vi "Read_Write_Plot_Setup.vi"(6 "jobDirectory":path, 7 "Mode":enum16{"Load", "Save"}(ring), 9 "Setup filename":string, 11 "Cluster":T1={"Result files to read"=[], "Template"=path "", "Transpose"=FALSE, "Additional X Values"=[], "Additional Y Values"=[], "Output Filename"=path "", "Create Picture Vi Name"="Intensity plot jpg.vi", "Intensity Plot?"=FALSE, "Multi Ordinate"=[], "Abscissa String"="", "Filter Array"=["", "", "", "", "", ""], "Filter Bins 1 Strings"=[""], "Filter Bins 2 Strings"=[""], "Filters 3 onwards"=[], "nRows"=0} {"Additional Y Values" format="%.2f"; "Additional X Values" format="%.2f"}) -> (0 "OK?":bool, 1 "setupLoaded":path, 3 "Cluster 2":T1={"Result files to read"=[], "Template"=path "", "Transpose"=FALSE, "Additional X Values"=[], "Additional Y Values"=[], "Output Filename"=path "", "Create Picture Vi Name"="Intensity plot jpg.vi", "Intensity Plot?"=FALSE, "Multi Ordinate"=[], "Abscissa String"="", "Filter Array"=["", "", "", "", "", ""], "Filter Bins 1 Strings"=[""], "Filter Bins 2 Strings"=[""], "Filters 3 onwards"=[], "nRows"=0} {"Additional Y Values" format="%.2f"; "Additional X Values" format="%.2f"})   [LabVIEW 2022 SP3]
uses:
  All_Setup.ctl
  File/Setup_Filetype.ctl
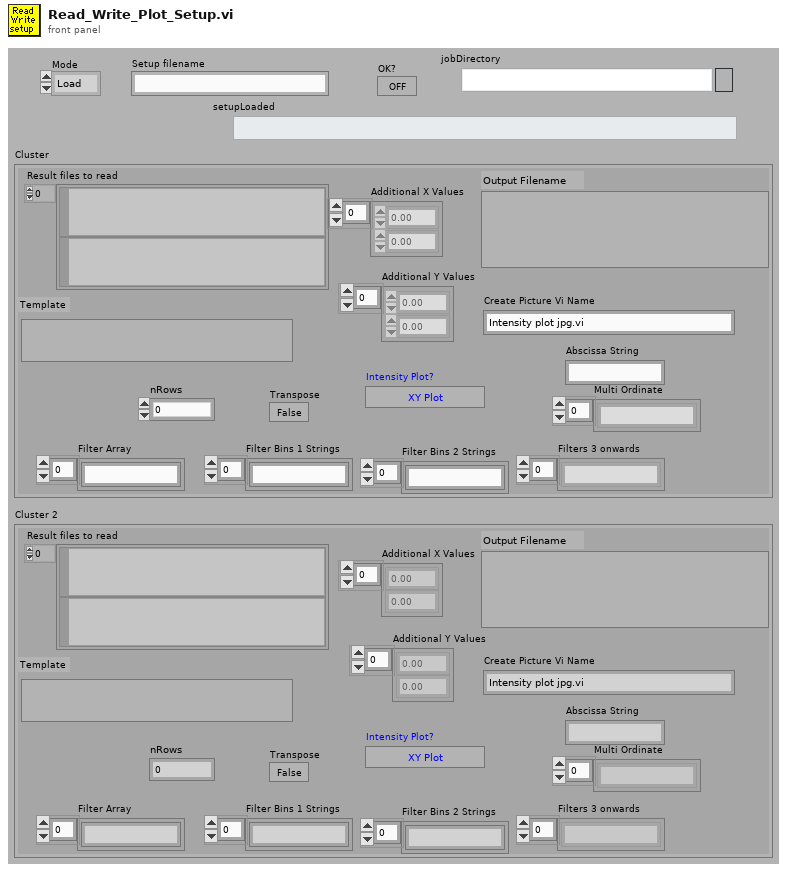
[diagram p1: front panel]
types:
  T1 = typedef "All_Setup.ctl" = cluster{"Result files to read":path[], "Template":path, "Transpose":bool, "Additional X Values":dbl[], "Additional Y Values":dbl[], "Output Filename":path, "Create Picture Vi Name":string, "Intensity Plot?":bool, "Multi Ordinate":string[], "Abscissa String":string, "Filter Array":string[], "Filter Bins 1 Strings":string[], "Filter Bins 2 Strings":string[], "Filters 3 onwards":string[], "nRows":i32}
  T2 = typedef "Setup_Filetype.ctl" = enum16{"Measurement Setups", "Calibration Setups", "General", "Results File Plotter Setups", "Speed Calib Tweaks"}
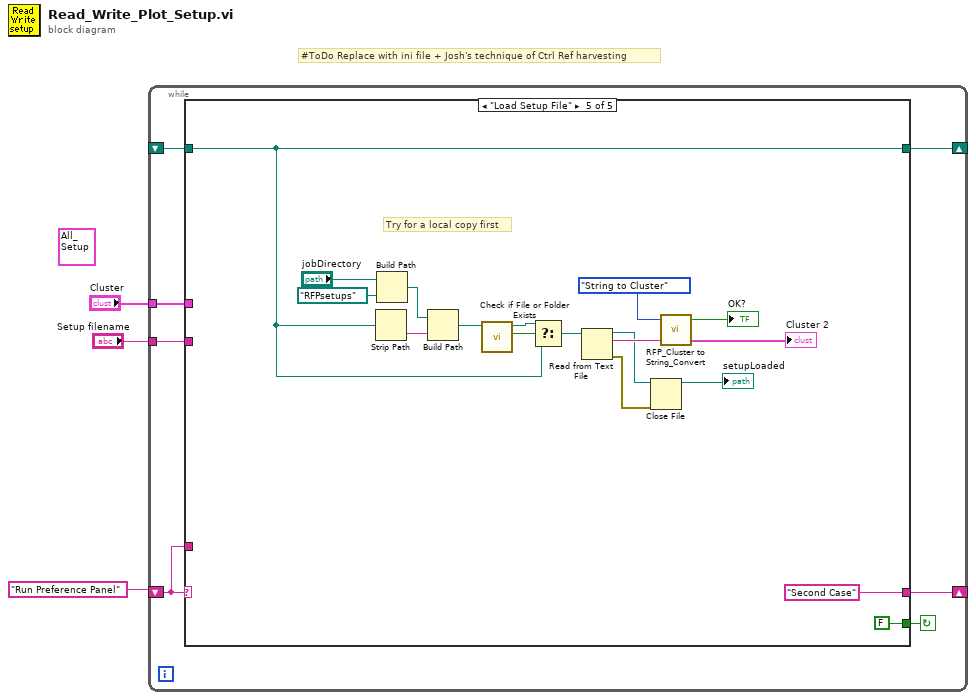
[diagram p0: block diagram]
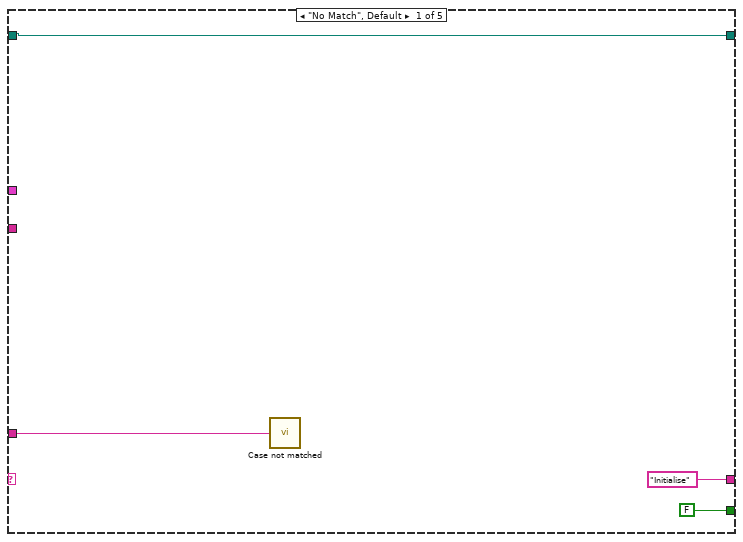
[diagram p2: hidden frame]
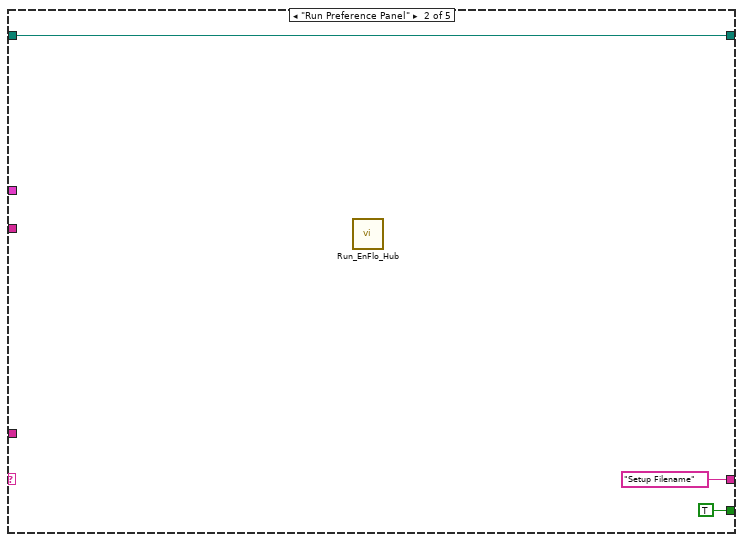
[diagram p3: hidden frame]
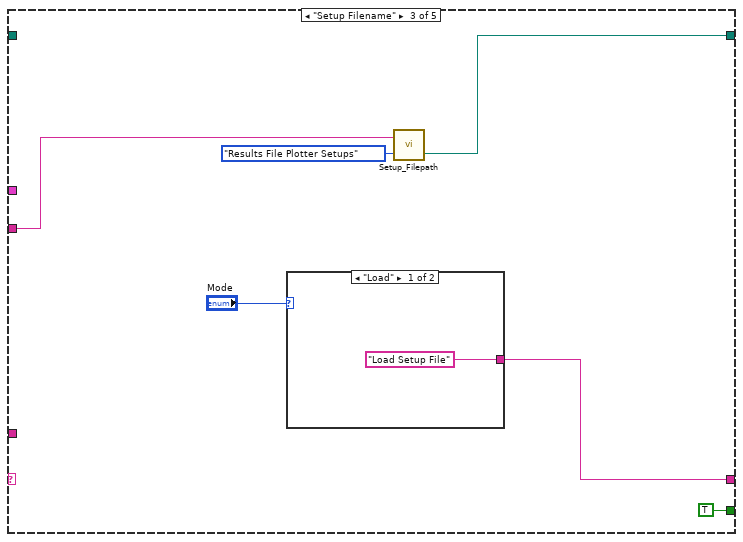
[diagram p4: hidden frame]
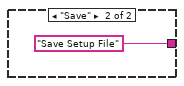
[diagram p5: hidden frame]
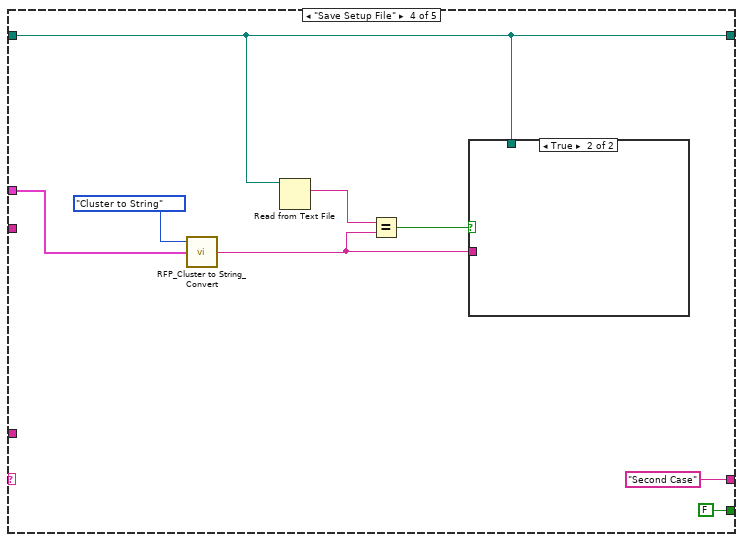
[diagram p6: hidden frame]
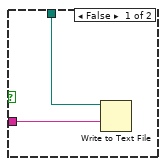
[diagram p7: hidden frame]
diagram:
  (unwired) T1 {"Result files to read"=[], "Template"=path "", "Transpose"=FALSE, "Additional X Values"=[], "Additional Y Values"=[], "Output Filename"=path "", "Create Picture Vi Name"="Intensity plot jpg.vi", "Intensity Plot?"=FALSE, "Multi Ordinate"=[], "Abscissa String"="", "Filter Array"=["", "", "", "", "", ""], "Filter Bins 1 Strings"=[""], "Filter Bins 2 Strings"=[""], "Filters 3 onwards"=[], "nRows"=0} ("Cluster")
  # "#ToDo Replace with ini file + Josh's technique of Ctrl Ref harvesting"
  n1 = while {
    shift-left: "Run Preference Panel" -> [w8]
    shift-right: [w9] -> _
    shift-right: [w6] -> _
    shift-left: _ -> [w7]
    tunnel: "Cluster" -> [w5]
    tunnel: "Setup filename" -> [w4]
    stop <- w10 continue-if-true
    n2 = case shown="\"Load Setup File\"" w8 {
      tunnel: [FALSE TRUE TRUE FALSE FALSE] -> w10
      tunnel: ["Initialise" "Setup Filename" w21 "Second Case" "Second Case"] -> w9
      tunnel: w8 -> [w11 _ _ _ _]
      tunnel: w7 -> [w12 w15 _ w30 w40]
      tunnel: [w12 w15 w18 w30 w40] -> w6
      tunnel: w5 -> [_ _ _ w31 _]
      tunnel: w4 -> [_ _ w19 _ _]
      frame "No Match", Default {
        n3 = call "Case not matched.vi"("Case Name not Matched"=w11) -> ()
      }
      frame "Run Preference Panel" {
        n4 = call "Run_EnFlo_Hub.vi"() -> ()  [unwired: 1 in, 7 out]
      }
      frame "Setup Filename" {
        n5 = case shown="\"Load\"" "Mode" {
          tunnel: ["Load Setup File" "Save Setup File"] -> w21
          frame "Load" {
          }
          frame "Save" {
          }
        }
        n6 = call "Setup_Filepath.vi"("Setup File Type"=Setup_Filetype."Results File Plotter Setups", "Filename in"=w19) -> ("Filename Out"=w18:path)  [unwired: 1 out]
      }
      frame "Save Setup File" {
        n7 = call "RFP_Cluster to String_Convert.vi"("Setup Cluster In"=w31, "Mode"=enum16{"Cluster to String", "String to Cluster"}."Cluster to String") -> ("Setup String Out"=w28:string)  [unwired: 1 in, 2 out]
        n8 = Read from Text File(file (use dialog)=w30) -> (text=w29:string)  [unwired: 3 in, 3 out]
        n9 = Equal?(x=w29, y=w28) -> (x = y?=w27:bool)
        n10 = case shown="True" w27 {
          tunnel: w30 -> [w35 _]
          tunnel: w28 -> [w34 _]
          frame False {
            n11 = Write to Text File(file (use dialog)=w35, text=w34) -> ()  [unwired: 2 in, 3 out]
          }
          frame True {
          }
        }
      }
      frame "Load Setup File" {
        # "Try for a local copy first"
        n12 = Strip Path(path=w40) -> (name=w45:string)  [unwired: 1 out]
        n13 = Build Path(base path="jobDirectory", name or relative path=path "RFPsetups") -> (appended path=w37:path)
        n14 = Build Path(base path=w37, name or relative path=w45) -> (appended path=w42:path)
        n15 = call <vilib>:"Check if File or Folder Exists.vi"("path"=w42) -> ("file or folder exists?"=w47:bool, "dup path"=w41:path)  [unwired: 8 in, 1 out]
        n16 = Select(t=w41, s=w47, f=w40) -> (s? t:f=w46:path)
        n17 = Read from Text File(file (use dialog)=w46) -> (refnum out=w44:refnum<file>, text=w50:string, error out=w43:errorcluster)  [unwired: 3 in, 1 out]
        n18 = Close File(refnum=w44, error in=w43) -> (path=→"setupLoaded":path)  [unwired: 1 out]
        n19 = call "RFP_Cluster to String_Convert.vi"("Setup String In"=w50, "Mode"=enum16{"Cluster to String", "String to Cluster"}."String to Cluster") -> ("Setup Cluster Out"=→"Cluster 2":T1, "OK?"=→"OK?":bool)  [unwired: 1 in, 1 out]
      }
    }
  }
